vi "SM motor repeat 2 tw.vi"(5 "Moving times":dbl, 6 "Waiting time (s)":dbl=3.0, 7 "Stop motion":bool, 8 "Move":bool, 9 "SM setting":T2={"Acceleration (mm/sec^2)"=1000.0, "Velocity (mm/sec)"=1.0, "Position (mm)"=0.0} {"Position (mm)" format="%.3f"; "Velocity (mm/sec)" format="%.3f"; "Acceleration (mm/sec^2)" format="%.3f"}, 10 "SM Config":T3={"VISA Serial ref"="COM3", "Motor Config"={"DriveRatio (mm/rev)"=10.16, "PosLimit + (mm)"=200.0, "PosLimit - (mm)"=0.0, "EncoderRatio (count/rev)"=2000.0, "MotorType"=enum."SM17"}} {"Motor Config"."EncoderRatio (count/rev)" format="%.2f"; "Motor Config"."PosLimit - (mm)" format="%.3f"; "Motor Config"."PosLimit + (mm)" format="%.3f"; "Motor Config"."DriveRatio (mm/rev)" format="%.2f"}) -> (1 "Status":T1, 3 "Position (mm)":dbl)   [LabVIEW 2015]
uses:
  magnetometers/smi/labview/CPM20Software/SmartMotor.llb/SM Config.ctl
  magnetometers/smi/labview/CPM20Software/SmartMotor.llb/SM MotorConfig.ctl
  magnetometers/smi/labview/CPM20Software/SmartMotor.llb/SM Status.ctl
  Global vab.vi
panel:
  out "Ccurrent times":dbl
  in  "Action":bool
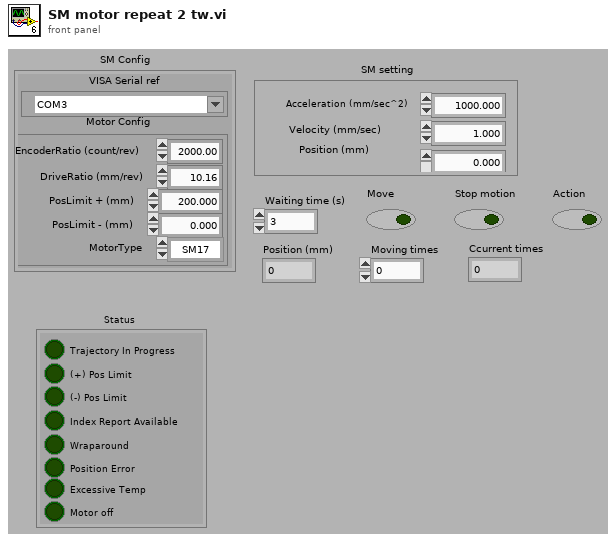
[diagram p1: front panel]
types:
  T1 = typedef "SM Status.ctl" = cluster{"Trajectory In Progress":bool, "(+) Pos Limit":bool, "(-) Pos Limit":bool, "Index Report Available":bool, "Wraparound":bool, "Position Error":bool, "Excessive Temp":bool, "Motor off":bool}
  T2 = cluster{"Acceleration (mm/sec^2)":dbl, "Velocity (mm/sec)":dbl, "Position (mm)":dbl}
  T3 = typedef "SM Config.ctl" = cluster{"VISA Serial ref":refnum<visa-resource-name>, "Motor Config":T4}
  T4 = typedef "SM MotorConfig.ctl" = cluster{"DriveRatio (mm/rev)":dbl, "PosLimit + (mm)":dbl, "PosLimit - (mm)":dbl, "EncoderRatio (count/rev)":dbl, "MotorType":enum16{"SM17", "SM23", "SM34", "SM42", "SM56"}}
  T5 = cluster{"Acceleration (mm/sec^2)":dbl, "Velocity (mm/sec)":dbl, "PosLimit - (mm)":dbl}
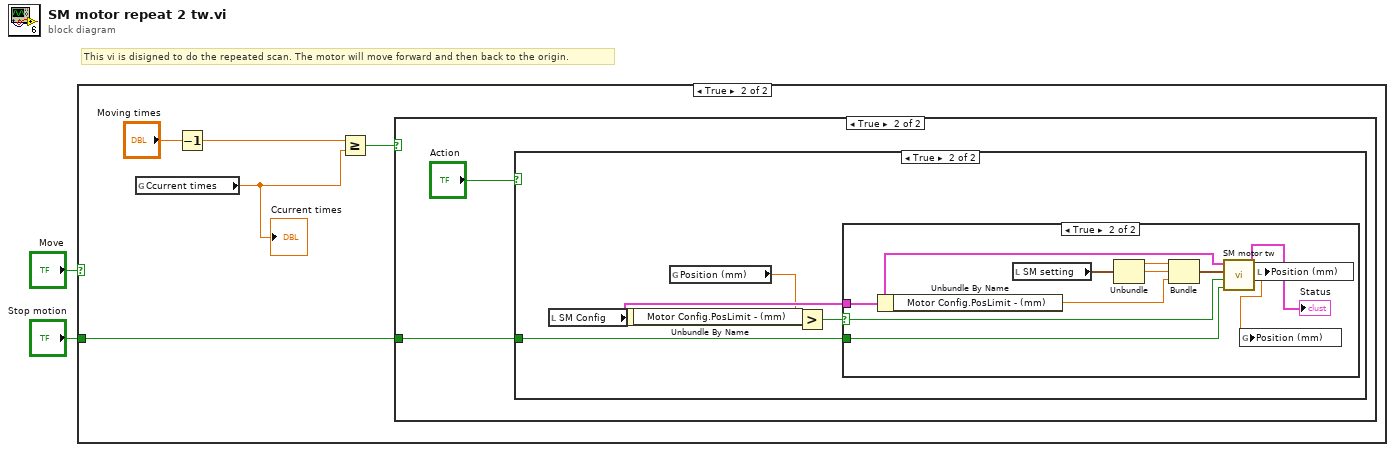
[diagram p0: block diagram]
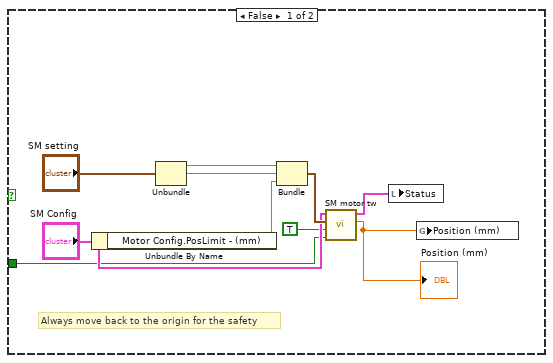
[diagram p2: hidden frame]
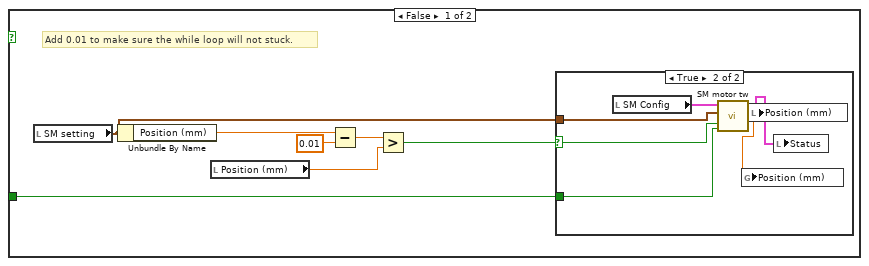
[diagram p4: hidden frame]
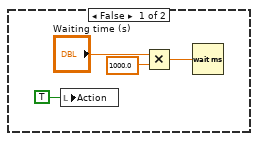
[diagram p5: hidden frame]
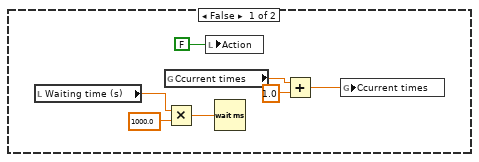
[diagram p6: hidden frame]
diagram:
  # "This vi is disigned to do the repeated scan. The motor will move forward and then back to the origin."
  n1 = case shown="True" "Move" {
    tunnel: "Stop motion" -> [w5 w15]
    frame False {
      # "Always move back to the origin for the safety"
      n2 = Unbundle By Name("SM Config") -> ("Motor Config.PosLimit - (mm)"=w9:dbl)
      n3 = Unbundle("SM setting") -> ("Acceleration (mm/sec^2)"=w12:dbl, "Velocity (mm/sec)"=w11:dbl)  [unwired: 1 out]
      n4 = Bundle("Acceleration (mm/sec^2)"=w12, "Velocity (mm/sec)"=w11, "PosLimit - (mm)"=w9) -> (w10:T5)  [unwired: 1 out]
      n5 = call "SM motor tw.vi"("SM Config"="SM Config", "SM setting"=w10, "Move"=TRUE, "Stop motion"=w5) -> ("Status"=w3:T1, "Position (mm)"=w4:dbl)  [unwired: 5 out]
      "Position (mm)" <- w4
      n6 = local write "Status"(w3) -> ()
      n7 = global write "Global vab.vi" "Position (mm)"(w4) -> ()
    }
    frame True {
      n8 = global read "Global vab.vi" "Ccurrent times"() -> (w13:dbl)
      "Ccurrent times" <- w13
      n9 = Decrement(x="Moving times") -> (x-1=w14:dbl)
      n10 = Greater Or Equal?(x=w14, y=w13) -> (x >= y?=w16:bool)
      n11 = case shown="True" w16 {
        tunnel: w15 -> [_ w19]
        frame False {
        }
        frame True {
          n12 = case shown="True" "Action" {
            tunnel: w19 -> [w21 w38]
            frame False {
              # "Add 0.01 to make sure the while loop will not stuck."
              n13 = local read "SM setting"() -> (w22:T2)
              n14 = Unbundle By Name(w22) -> ("Position (mm)"=w25:dbl)
              n15 = local read "Position (mm)"() -> (w20:dbl)
              n16 = Subtract(x=w25, y=0.01) -> (x-y=w24:dbl)
              n17 = Greater?(x=w24, y=w20) -> (0:w23:bool)
              n18 = case shown="True" w23 {
                selector: w23 -> [_ w34]
                tunnel: w22 -> [_ w35]
                tunnel: w21 -> [_ w33]
                frame False {
                  n19 = local write "Action"(TRUE ("Action")) -> ()
                  n20 = Multiply(x="Waiting time (s)", y=1000.0) -> (x*y=w30:dbl)
                  n21 = Wait (ms)(milliseconds to wait=w30) -> ()  [unwired: 1 out]
                }
                frame True {
                  n22 = local read "SM Config"() -> (w36:T3)
                  n23 = call "SM motor tw.vi"("SM Config"=w36, "SM setting"=w35, "Move"=w34, "Stop motion"=w33) -> ("Status"=w31:T1, "Position (mm)"=w32:dbl)  [unwired: 5 out]
                  n24 = global write "Global vab.vi" "Position (mm)"(w32) -> ()
                  n25 = local write "Position (mm)"(w32) -> ()
                  n26 = local write "Status"(w31) -> ()
                }
              }
            }
            frame True {
              n27 = local read "SM Config"() -> (w40:T3)
              n28 = Unbundle By Name(w40) -> ("Motor Config.PosLimit - (mm)"=w39:dbl)
              n29 = global read "Global vab.vi" "Position (mm)"() -> (w37:dbl)
              n30 = Greater?(x=w37, y=w39) -> (0:w41:bool)
              n31 = case shown="True" w41 {
                selector: w41 -> [_ w53]
                tunnel: w40 -> [_ w52]
                tunnel: w38 -> [_ w51]
                frame False {
                  n32 = local read "Waiting time (s)"() -> (w42:dbl)
                  n33 = global read "Global vab.vi" "Ccurrent times"() -> (w45:dbl)
                  n34 = Multiply(x=w42, y=1000.0) -> (x*y=w43:dbl)
                  n35 = local write "Action"(FALSE ("Action")) -> ()
                  n36 = Wait (ms)(milliseconds to wait=w43) -> ()  [unwired: 1 out]
                  n37 = Add(x=w45, y=1.0) -> (x+y=w46:dbl)
                  n38 = global write "Global vab.vi" "Ccurrent times"(w46) -> ()
                }
                frame True {
                  n39 = Unbundle By Name(w52) -> ("Motor Config.PosLimit - (mm)"=w57:dbl)
                  n40 = local read "SM setting"() -> (w54:T2)
                  n41 = Unbundle(w54) -> ("Acceleration (mm/sec^2)"=w55:dbl, "Velocity (mm/sec)"=w56:dbl)  [unwired: 1 out]
                  n42 = Bundle("Acceleration (mm/sec^2)"=w55, "Velocity (mm/sec)"=w56, "PosLimit - (mm)"=w57) -> (w58:T5)  [unwired: 1 out]
                  n43 = call "SM motor tw.vi"("SM Config"=w52, "SM setting"=w58, "Move"=w53, "Stop motion"=w51) -> ("Status"=→"Status":T1, "Position (mm)"=w50:dbl)  [unwired: 5 out]
                  n44 = global write "Global vab.vi" "Position (mm)"(w50) -> ()
                  n45 = local write "Position (mm)"(w50) -> ()
                }
              }
            }
          }
        }
      }
    }
  }
